vi "Read commandName.vi"(8 "error in (no error)":errorcluster, 11 "Exit in":refnum<class "Exit.lvclass">) -> (0 "error out":errorcluster, 2 "CommandValue":T1, 3 "Exit out":refnum<class "Exit.lvclass">)   [LabVIEW 2016, in "Commands.lvlib" / "Exit.lvclass"]
uses:
  Exit.lvclass
  Typedefs/CommandValue.ctl
  Typedefs/EXATypedefs.lvlib
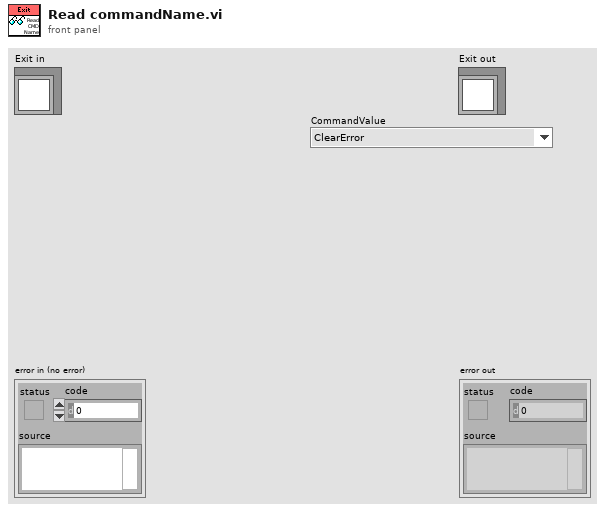
[diagram p1: front panel]
types:
  T1 = typedef "EXATypedefs.lvlib/CommandValue.ctl" = enum16{"ClearError", "Disable", "Enable", "Exit", "GoToStandby", "OnHeartbeat", "OnIncomingMessagingError", "OnInterrupt", "Start"}
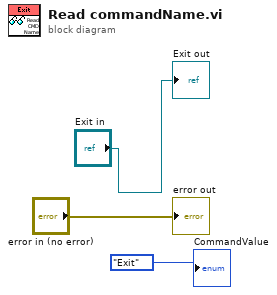
[diagram p0: block diagram]
diagram:
  "error out" <- "error in (no error)"
  "Exit out" <- "Exit in"
  "CommandValue" <- CommandValue."Exit" ("CommandValue")
